vi "niFPGA BW CU Order 1 (16-bit).vi"(0 "filter state in":i16, 1 "reset":bool, 5 "input data":i16, 7 "accumulator in":i32, 9 "adder in":i32, 11 "iteration":u8, 12 "in shift":i8=-1, 13 "lowpass?":bool) -> (4 "filter state out":i16, 6 "multiplier":i32, 8 "accumulator out":i32, 10 "adder out":i32, 15 "terminate":bool)   [LabVIEW 2017]
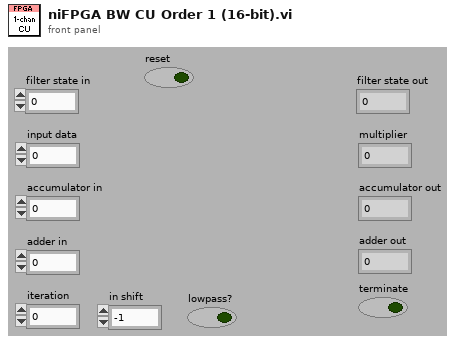
[diagram p1: front panel]
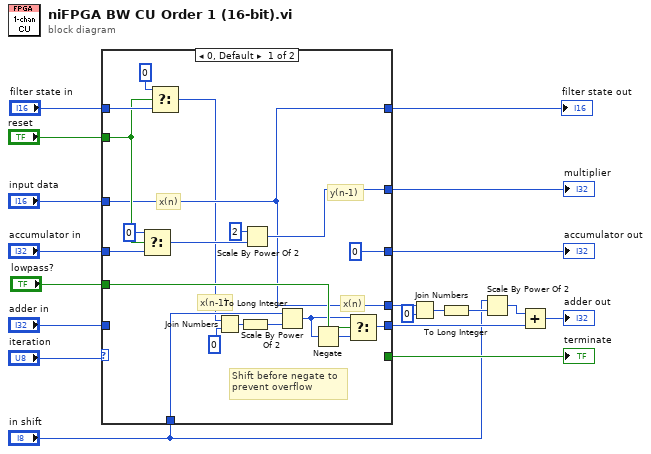
[diagram p0: block diagram]
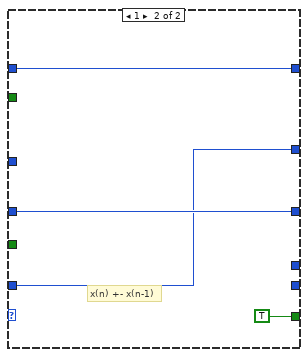
[diagram p2: hidden frame]
diagram:
  n1 = case shown="0, Default" "iteration" {
    tunnel: [w24 w41] -> w11
    tunnel: "input data" -> [w24 _]
    tunnel: [w20 _] -> w8
    tunnel: "adder in" -> [_ w40]
    tunnel: [w27 w40] -> w10
    tunnel: [w24 _] -> w7
    tunnel: [0 ("Numeric") w42] -> w9
    tunnel: [_ TRUE] -> w6
    tunnel: "reset" -> [w30 _]
    tunnel: "accumulator in" -> [w32 w42]
    tunnel: "filter state in" -> [w31 w41]
    tunnel: "in shift" -> [w25 _]
    tunnel: "lowpass?" -> [w28 _]
    frame 0, Default {
      # "Shift before negate to\nprevent overflow"
      # "x(n)"
      # "x(n-1)"
      # "x(n)"
      # "y(n-1)"
      n2 = Select(t=0, s=w30, f=w32) -> (s? t:f=w33:i32)
      n3 = Select(t=i16 0 ("filter state in"), s=w30, f=w31) -> (s? t:f=w23:i16)
      n4 = Join Numbers(hi=w23, lo=i16 0) -> ((hi.lo)=w38:u32)
      n5 = To Long Integer(number=w38) -> (32bit integer=w22:i32)
      n6 = Scale By Power Of 2(n=2, x=w33) -> (x*2^n=w27:i32)
      n7 = Scale By Power Of 2(n=w25, x=w22) -> (x*2^n=w21:i32)
      n8 = Negate(x=w21) -> (-x=w29:i32)
      n9 = Select(t=w21, s=w28, f=w29) -> (s? t:f=w20:i32)
    }
    frame 1 {
      # "x(n) +- x(n-1)"
    }
  }
  "multiplier" <- w10
  "terminate" <- w6
  "accumulator out" <- w9
  "filter state out" <- w11
  n10 = Join Numbers(hi=w7, lo=i16 0) -> ((hi.lo)=w18:u32)
  n11 = To Long Integer(number=w18) -> (32bit integer=w17:i32)
  n12 = Scale By Power Of 2(n="in shift", x=w17) -> (x*2^n=w19:i32)
  n13 = Add(x=w19, y=w8) -> (x+y=→"adder out":i32)
